vi "TC test USB4718 v2.vi"() -> ()   [LabVIEW 2013]
uses:
  <vilib>/Platform/TimedLoop/XDataNode/timing_clust.ctl
  <vilib>/Platform/TimedLoop/XDataNode/nitl_modes.ctl
  <vilib>/Platform/TimedLoop/XDataNode/wakeup.ctl
  <vilib>/platform/TimedLoop/XDataNode/XDataNode.xnode
  <vilib>/Platform/TimedLoop/XDataNode/XDNodeRunTimeDep.lvlib
panel:
  in  "Stop & Open File":bool
  out "Waveform Chart":dynamicdata(graph)
  out "data file":string
  out "tdms file out":refnum<k34>
  out "CYCLES":dbl
  out "cycle":bool
  out "T3":dbl
  out "T2":dbl
  out "T1":dbl
  out "T0":dbl
  # "Note: Use ABORT button to stop program without displaying data file."
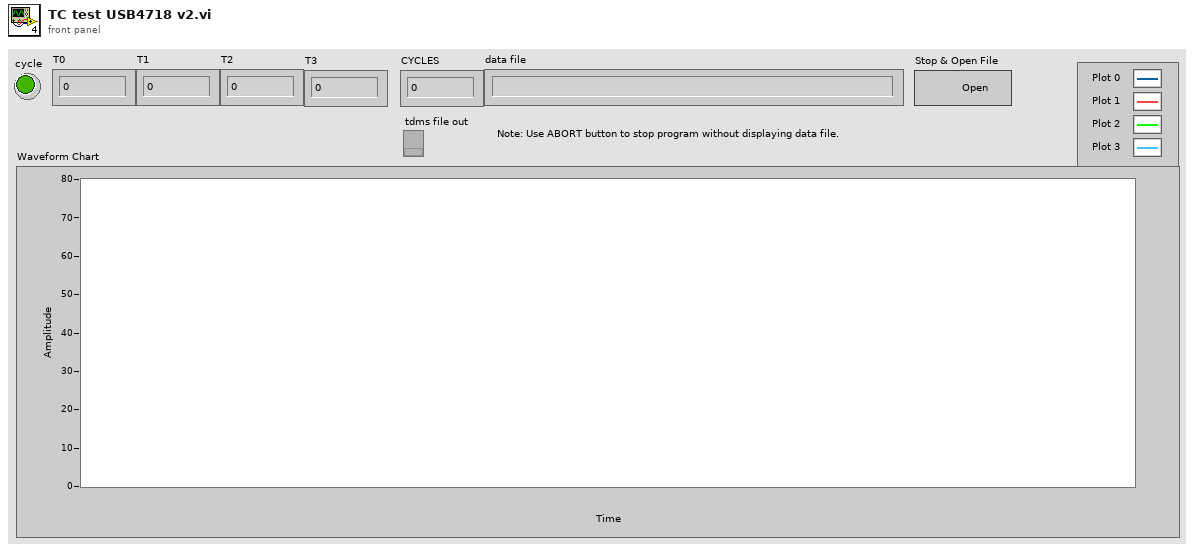
[diagram p1: front panel]
types:
  T1 = enum16{"open", "open or create", "create or replace", "create", "open (read-only)"}
  T2 = typedef "XDNodeRunTimeDep.lvlib/timing_clust.ctl" = cluster{"Expected End [f-1]":u64, "Actual End [f-1]":u64, "Finished Late? [f-1]":bool, "Expected End [i-1]":u64, "Actual End [i-1]":u64, "Finished Late? [i-1]":bool, "Expected Start [i]":u64, "Actual Start [i]":u64, "Expected Start [f]":u64, "Actual Start [f]":u64, "Source Name":string, "Structure Name":string, "Period":i64, "Deadline":i64, "Offset":i64, "Start":i64, "Priority":i32, "Timeout":i32, "Mode":T3, "Wakeup Reason":T4, "Error":errorcluster, "Source Type":string, "Secondary Source Type":string, "Global End Time":u64, "Global Start Time":u64, "Frame Duration":u64, "Iteration Duration":u64, "Assigned CPU":i32, "I/O Scan Engine Mode":u32}
  T3 = typedef "XDNodeRunTimeDep.lvlib/nitl_modes.ctl" = enum32{"No Change", "Process missed periods, maintain original phase", "Discard missed periods, maintain original phase", "Process missed periods, ignore original phase", "Discard missed periods, ignore original phase"}
  T4 = typedef "XDNodeRunTimeDep.lvlib/wakeup.ctl" = enum32{"Normal", "Aborted", "Asynchronous wakeup", "Timing source error", "Timed loop error", "Timeout"}
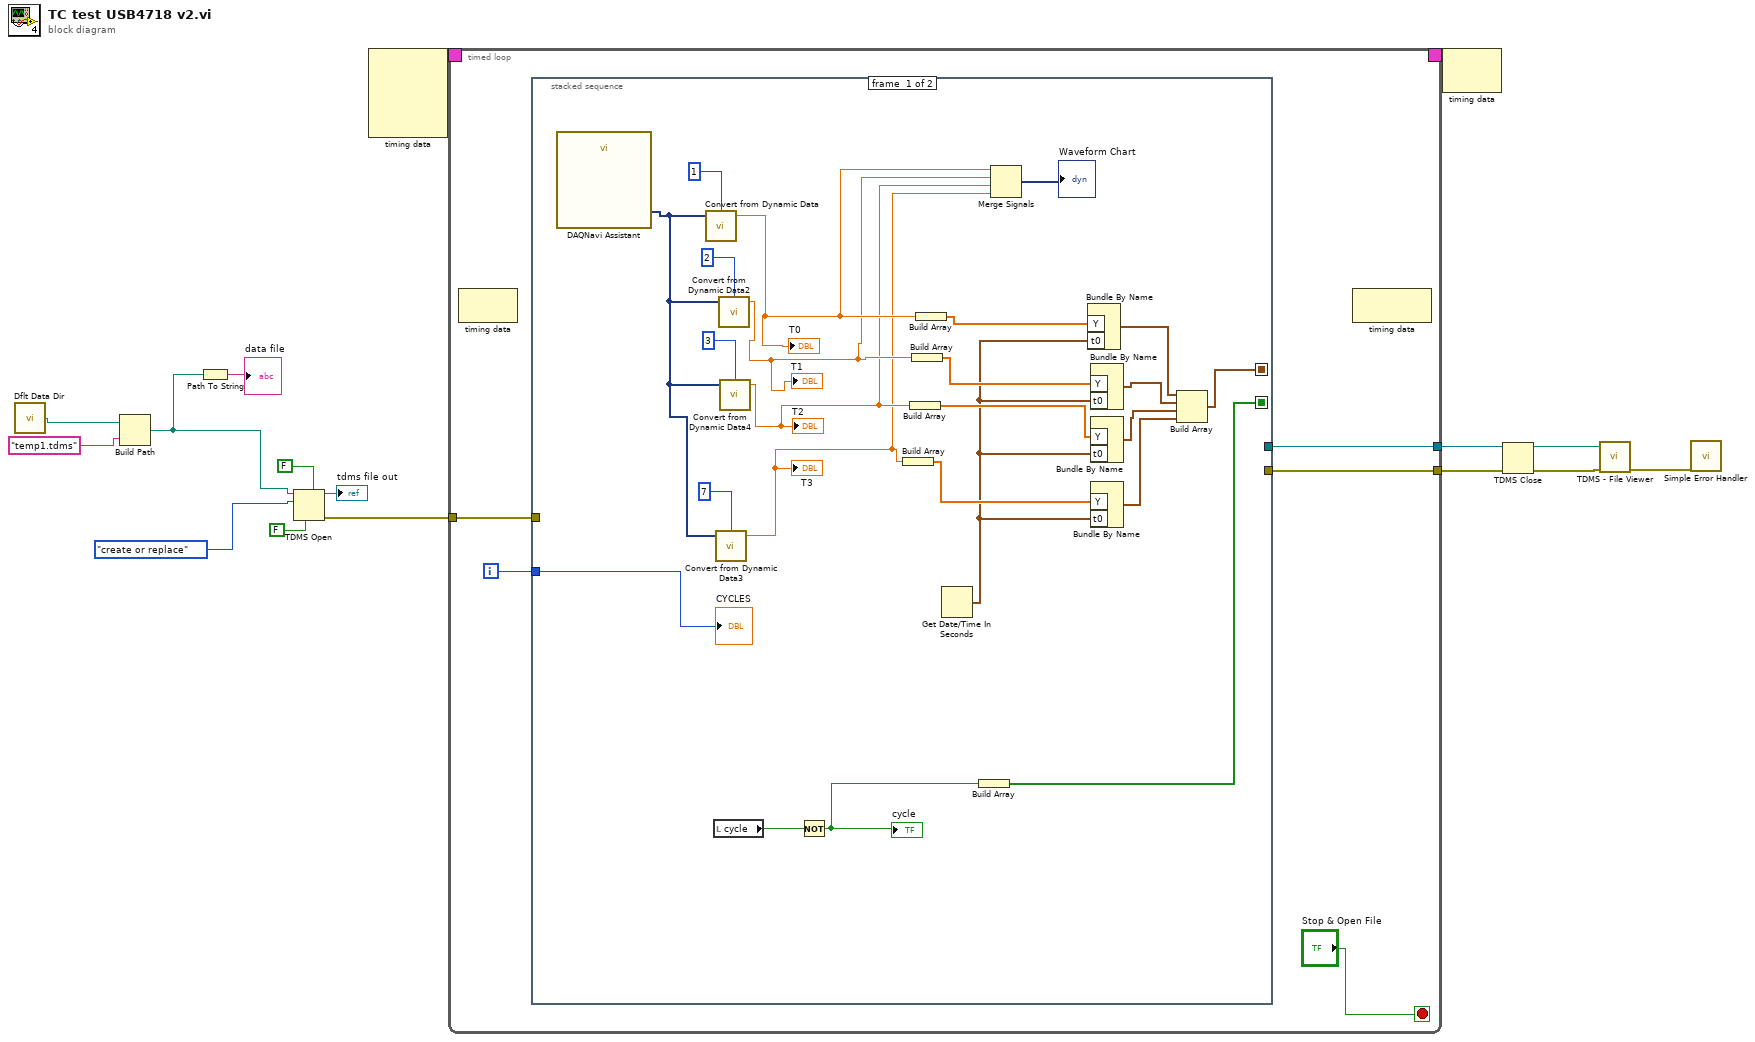
[diagram p0: block diagram]
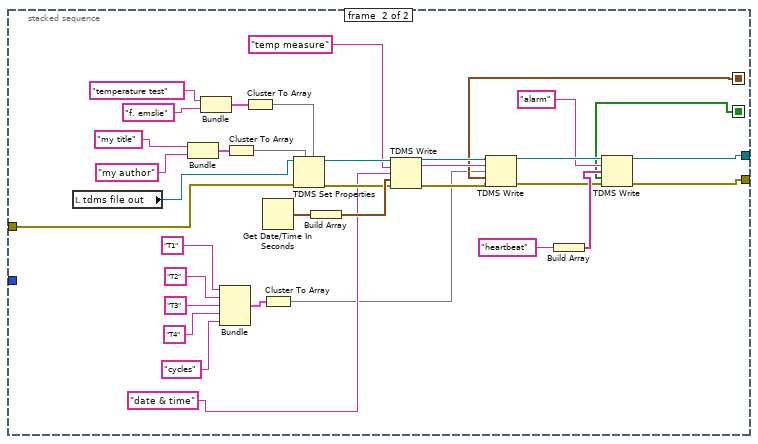
[diagram p2: hidden frame]
diagram:
  n1 = call <vilib>:"Dflt Data Dir.vi"() -> ("App:Default Data Directory"=w4:path)
  n2 = Build Path(base path=w4, name or relative path="temp1.tdms") -> (appended path=w5:path)
  n3 = Path To String(path=w5) -> (string=→"data file":string)
  n4 = TDMS Open(5:FALSE ("create index file? (T)"), 6:FALSE ("disable buffering? (T)"), 10:T1."create or replace" ("operation (0:open)"), 11:w5) -> (0:w12:errorcluster, 3:→"tdms file out":refnum<k34>)  [unwired: 3 in]
  n5 = node-c288() -> (w16:T2)  [unwired: 4 in]
  n6 = timed-loop {
    timing: w16 -> [_]
    timing-out: [_] -> w15
    tunnel: w12 -> [w20]
    tunnel: [w19] -> w11
    tunnel: [w18] -> w10
    i -> [w21]
    stop <- "Stop & Open File" stop-if-true
    n7 = node-c288() -> ()  [unwired: 1 in, 1 out]
    n8 = stacked-sequence {
      seq-local: [w36 _] -> [_ w56]
      seq-local: [w32 _] -> [_ w51]
      tunnel: w21 -> [w44 _]
      tunnel: w20 -> [_ w65]
      tunnel: [_ w49] -> w19
      tunnel: [_ w48] -> w18
      frame #0 {
        n9 = call "DAQNavi Assistant"() -> ("data out(DDT)"=w27:dynamicdata)  [unwired: 26 in, 1 out]
        n10 = call "Convert from Dynamic Data"("Dynamic Data Type"=w27, "Channel"=1) -> ("Scalar"=w25:dbl)  [unwired: 2 in]
        "T0" <- w25
        n11 = local read "cycle"() -> (w45:bool)
        n12 = call "Convert from Dynamic Data3"("Dynamic Data Type"=w27, "Channel"=7) -> ("Scalar"=w22:dbl)  [unwired: 2 in]
        "T3" <- w22
        n13 = call "Convert from Dynamic Data2"("Dynamic Data Type"=w27, "Channel"=2) -> ("Scalar"=w24:dbl)  [unwired: 2 in]
        "T1" <- w24
        n14 = call "Convert from Dynamic Data4"("Dynamic Data Type"=w27, "Channel"=3) -> ("Scalar"=w23:dbl)  [unwired: 2 in]
        "T2" <- w23
        n15 = Not(x=w45) -> (.not. x?=w43:bool)
        "cycle" <- w43
        n16 = Build Array(w22) -> (w39:dbl[])
        n17 = Build Array(w23) -> (w40:dbl[])
        n18 = Build Array(w24) -> (w41:dbl[])
        n19 = Build Array(w25) -> (w42:dbl[])
        n20 = Get Date/Time In Seconds() -> (seconds since 1Jan1904=w37:timestamp)
        n21 = Build Array(w43) -> (w32:bool[])
        n22 = Merge Signals(w25, w24, w23, w22) -> (→"Waveform Chart":dynamicdata)
        n23 = Bundle By Name("Y"=w42, "t0"=w37) -> (w38:waveform(dbl))  [unwired: 1 in]
        n24 = Bundle By Name("Y"=w41, "t0"=w37) -> (w35:waveform(dbl))  [unwired: 1 in]
        n25 = Bundle By Name("Y"=w40, "t0"=w37) -> (w34:waveform(dbl))  [unwired: 1 in]
        n26 = Bundle By Name("Y"=w39, "t0"=w37) -> (w33:waveform(dbl))  [unwired: 1 in]
        n27 = Build Array(w38, w35, w34, w33) -> (w36:waveform(dbl)[])
        "CYCLES" <- w44
      }
      frame #1 {
        n28 = local read "tdms file out"() -> (w47:refnum<k34>)
        n29 = Bundle("my title", "my author") -> (w68:cluster{string, string})  [unwired: 1 in]
        n30 = Bundle("temperature test", "f. emslie") -> (w71:cluster{string, string})  [unwired: 1 in]
        n31 = Bundle("T1", "T2", "T3", "T4", "cycles") -> (w76:cluster{string, string, string, string, string})  [unwired: 1 in]
        n32 = Cluster To Array(cluster=w68) -> (array=w69:string[])
        n33 = Cluster To Array(cluster=w71) -> (array=w67:string[])
        n34 = Get Date/Time In Seconds() -> (seconds since 1Jan1904=w74:timestamp)
        n35 = Cluster To Array(cluster=w76) -> (array=w46:string[])
        n36 = TDMS Set Properties(5:w67, 7:w69, 8:w65, 11:w47) -> (0:w63:errorcluster, 3:w62:refnum<k34>)  [unwired: 2 in, 2 out]
        n37 = Build Array(w74) -> (w64:timestamp[])
        n38 = TDMS Write(0:w62, 5:"temp measure", 7:"date & time", 9:w64, 11:w63) -> (4:w58:refnum<k34>, 6:w57:string, 15:w59:errorcluster)  [unwired: 1 in, 1 out]
        n39 = TDMS Write(0:w58, 5:w57, 7:w46, 9:w56, 11:w59) -> (4:w55:refnum<k34>, 15:w50:errorcluster)  [unwired: 1 in, 2 out]
        n40 = Build Array("heartbeat") -> (w52:string[])
        n41 = TDMS Write(0:w55, 5:"alarm", 7:w52, 9:w51, 11:w50) -> (4:w49:refnum<k34>, 15:w48:errorcluster)  [unwired: 1 in, 2 out]
      }
    }
    n42 = node-c288() -> ()  [unwired: 1 in, 1 out]
  }
  n43 = node-c288(w15) -> ()  [unwired: 1 out]
  n44 = TDMS Close(8:w10, 11:w11) -> (0:w3:errorcluster, 3:w1:path)
  n45 = call <vilib>:"TDMS - File Viewer.vi"("error in (no error)"=w3, "file path"=w1) -> ("error out"=w2:errorcluster)  [unwired: 4 in, 1 out]
  n46 = call <vilib>:"Simple Error Handler.vi"("error in (no error)"=w2) -> ()  [unwired: 4 in, 5 out]
